vi "GetSubPanelVIName [Wrapper].vi"(0 "Application in":refnum<vi>, 5 "VI Name":string, 7 "SubPanel Label":string, 11 "error in (no error)":errorcluster) -> (4 "Application out":refnum<vi>, 6 "VI Name":string, 15 "error out":errorcluster)   [LabVIEW 2016]
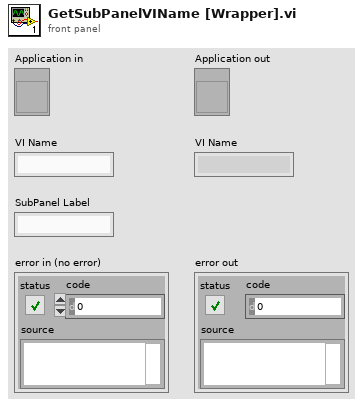
[diagram p1: front panel]
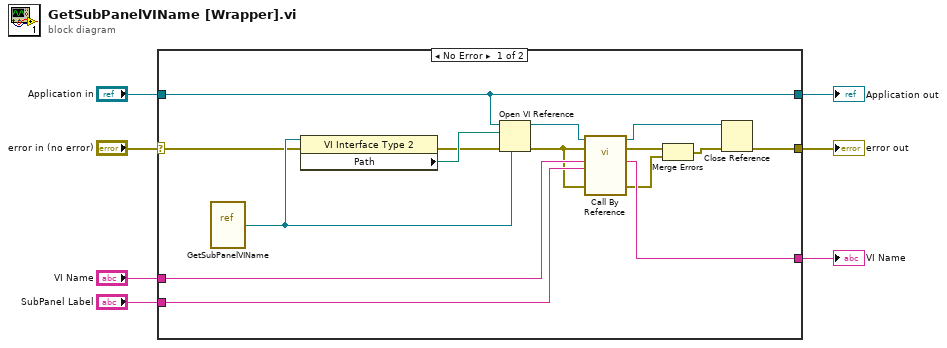
[diagram p0: block diagram]
diagram:
  n1 = case shown="No Error" "error in (no error)" {
    selector: "error in (no error)" -> [w13 w24]
    tunnel: "Application in" -> [w8 w23]
    tunnel: "VI Name" -> [w20 _]
    tunnel: [w19 _] -> w5
    tunnel: "SubPanel Label" -> [w18 _]
    tunnel: [w11 w24] -> w2
    tunnel: [w8 w23] -> w1
    frame No Error {
      n2 = vi-ref "GetSubPanelVIName.vi"() -> (w21:refnum<vi>)
      n3 = property class="VI Interface Type 2"(reference=w21, error in=w13) -> (error out=w14:errorcluster, "Path"=w22:path)  [unwired: 1 out]
      n4 = Open VI Reference(type specifier VI Refnum (for type only)=w21, application reference (local)=w8, vi path=w22, error in (no error)=w14) -> (vi reference=w15:refnum<vi>, error out=w12:errorcluster)  [unwired: 2 in]
      n5 = call-by-ref "?"(reference=w15, error in=w12, "VIName"=w20, "SubPanelLabel"=w18, 11:"error in (no error)"=w12) -> (reference out=w17:refnum<vi>, error out=w16:errorcluster, "VI Name"=w19:string, 15:"error out"=w9:errorcluster)  [unwired: 11 in]
      n6 = Merge Errors(w16, w9) -> (w10:errorcluster)
      n7 = Close Reference(reference=w17, error in (no error)=w10) -> (error out=w11:errorcluster)
    }
    frame Error {
    }
  }
  "error out" <- w2
  "VI Name" <- w5
  "Application out" <- w1
